vi "Write Channel Data with Headers.vi"() -> ()   [LabVIEW 2012]
uses:
  <vilib>/Analysis/NI_AALBase.lvlib
panel:
  in  "通道1名称":string="测试数据1"
  in  "通道0名称":string="测试数据2"
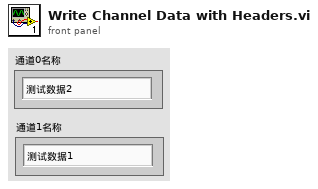
[diagram p1: front panel]
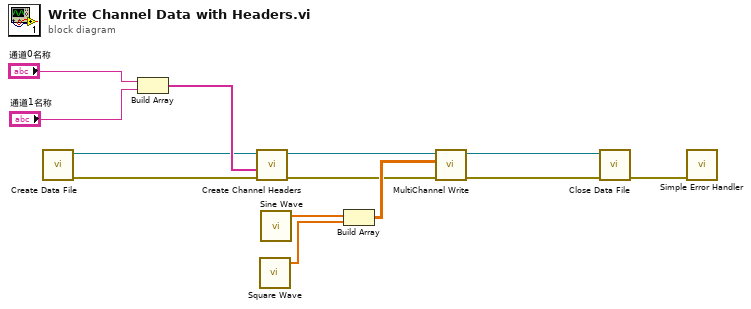
[diagram p0: block diagram]
diagram:
  n1 = call "Create Data File.vi"() -> ("错误输出"=w7:cluster{"状态":bool, "代码":i32, "源":string}, "文件引用句柄"=w6:refnum<file>)  [unwired: 10 in]
  n2 = Build Array ("创建数组")("通道0名称", "通道1名称") -> (w8:string[])
  n3 = call "Create Channel Headers.vi"("错误输入"=w7, "通道名"=w8, "文件引用句柄输入"=w6) -> ("错误输出"=w2:cluster{"状态":bool, "代码":i32, "源":string}, "文件引用句柄输出"=w5:refnum<file>)  [unwired: 7 in]
  n4 = call <vilib>:"Square Wave.vi"() -> ("square wave"=w11:dbl[])  [unwired: 6 in, 2 out]
  n5 = call <vilib>:"Sine Wave.vi"() -> ("sine wave"=w12:dbl[])  [unwired: 5 in, 2 out]
  n6 = Build Array ("创建数组")(w12, w11) -> (w3:dbl[][])
  n7 = call "MultiChannel Write.vi"("错误输入"=w2, "数据至记录"=w3, "文件引用句柄输入"=w5) -> ("错误输出"=w1:cluster{"状态":bool, "代码":i32, "源":string}, "文件引用句柄输出"=w4:refnum<file>)  [unwired: 7 in]
  n8 = call "Close Data File.vi"("错误输入"=w1, "文件引用句柄输入"=w4) -> ("错误输出"=w13:errorcluster)  [unwired: 9 in]
  n9 = call <vilib>:"Simple Error Handler.vi"("error in (no error)"=w13) -> ()  [unwired: 4 in, 5 out]
